vi "TX Message.vi"(8 "error in (no error)":errorcluster, 10 "variant":variant, 11 "Throttle Position in":refnum<class "Throttle Position.lvclass">) -> (0 "error out":errorcluster, 3 "Throttle Position out":refnum<class "Throttle Position.lvclass">)   [LabVIEW 2011, in "Throttle Position.lvclass"]
uses:
  Throttle Position.lvclass
  PID.lvclass
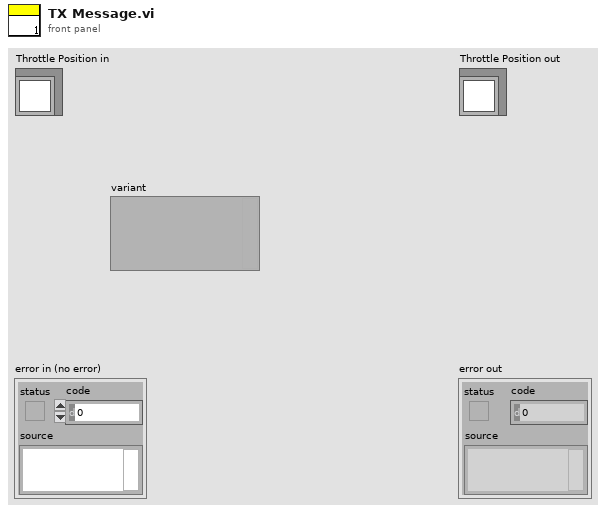
[diagram p1: front panel]
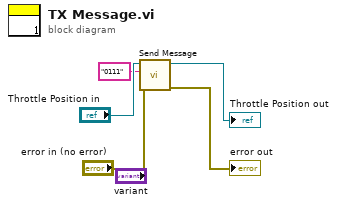
[diagram p0: block diagram]
diagram:
  n1 = call "Send Message.vi"("error in (no error)"="error in (no error)", "TX Message"="0111", "PID in"="Throttle Position in") -> ("error out"=→"error out":errorcluster, "PID out"=→"Throttle Position out":refnum<class "Throttle Position.lvclass">)  [unwired: 7 in]
